vi "fix all paths.vi"(11 "args":string[](array[string])) -> (2 "found":bool[](array[boolean]), 3 "paths out":path[](array[path]))   [LabVIEW 2016]
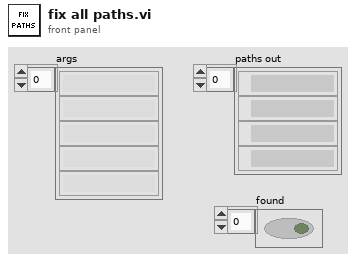
[diagram p1: front panel]
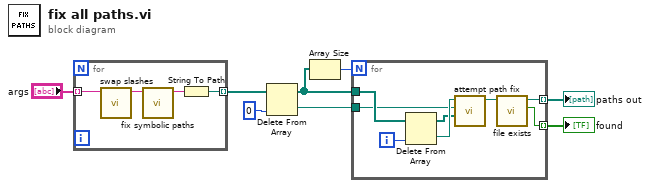
[diagram p0: block diagram]
diagram:
  n1 = for {
    tunnel: [w10] -> w2 mode=indexing
    tunnel: "args" -> [w9] mode=indexing
    n2 = call "swap slashes.vi"("in"=w9) -> ("out"=w12:string)  [unwired: 10 in]
    n3 = call "fix symbolic paths.vi"("in"=w12) -> ("out"=w11:string)  [unwired: 10 in]
    n4 = String To Path(string=w11) -> (path=w10:path)
  }
  n5 = Delete From Array(array=w2, index=0) -> (deleted portion=w3:path, array with subset deleted=w7:path[])  [unwired: 1 in]
  n6 = Array Size(array=w7) -> (size(s)=w6:i32)
  n7 = for {
    N: w6 -> [_]
    tunnel: w7 -> [w20]
    tunnel: w3 -> [w16]
    tunnel: [w14] -> w4 mode=indexing
    tunnel: [w13] -> w5 mode=indexing
    i -> [w19]
    n8 = Delete From Array(array=w20, index=w19) -> (deleted portion=w18:path, array with subset deleted=w17:path[])  [unwired: 1 in]
    n9 = call "attempt path fix.vi"("other possible paths"=w17, "working directory"=w16, "path to fix"=w18) -> ("path out"=w15:path)  [unwired: 8 in]
    n10 = call "file exists.vi"("Path in"=w15) -> ("file exists"=w13:bool, "Path out"=w14:path)  [unwired: 9 in]
  }
  "found" <- w5
  "paths out" <- w4
